vi "Global 1.vi"() -> ()   [LabVIEW 2011]
panel:
  in  "SAve USB Config":path
  in  "USB DAQ INI":path
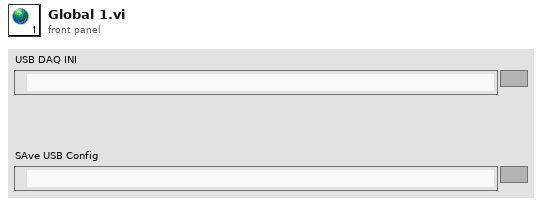
[diagram p1: front panel]
diagram:
